vi "GCliExit.vi"(8 "error in (no error)":errorcluster, 10 "No Error Code (0)":i32, 11 "CLI in":refnum<class "CLI.lvclass">) -> (0 "error out":errorcluster)   [LabVIEW 2023, in "CICD.lvlib"]
uses:
  CICD.lvlib
  <vilib>/Wiresmith Technology/G CLI/CLI Class/CLI.lvclass
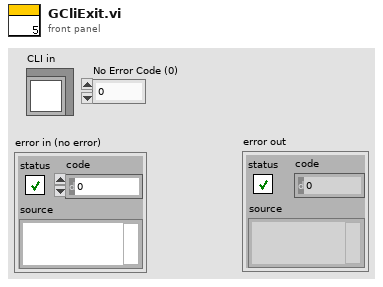
[diagram p1: front panel]
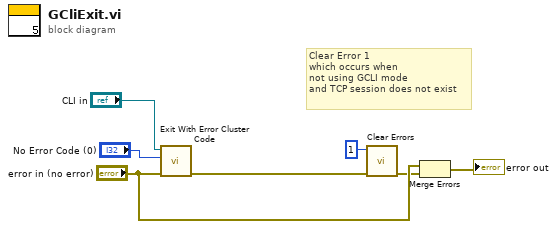
[diagram p0: block diagram]
diagram:
  # "Clear Error 1\nwhich occurs when\nnot using GCLI mode\nand TCP session does not exist"
  n1 = call <vilib>:"Exit With Error Cluster Code.vi"("error in (no error)"="error in (no error)", "No Error Code (0)"="No Error Code (0)", "CLI in"="CLI in") -> ("error out"=w6:errorcluster)  [unwired: 8 in]
  n2 = call <vilib>:"Clear Errors.vi"("error in (no error)"=w6, "specific error code to clear (0: all)"=1) -> ("error out"=w3:errorcluster)  [unwired: 4 in, 1 out]
  n3 = Merge Errors("error in (no error)", w3) -> (→"error out":errorcluster)
